vi "W7X2DPut_DAZ.vi"(4 "dimensions":i64[](array[numeric])=[1399090569999999999, -1], 5 "values":T1(array[cluster]), 6 "pulse_length":dbl, 7 "Unit":string, 8 "sample period":dbl, 9 "sample rate":u16, 10 "SigJSONbuffer":string, 11 "SigLabel":string) -> (0 "Parlog error out":errorcluster)   [LabVIEW 2014]
uses:
  <vilib>/httpClient/POSTBuffer.vi
  <vilib>/httpClient/LabVIEWHTTPClient.lvlib
panel:
  out "JSON string":string
  out "body":string
  out "headers":string
  out "body Parlog":string
  out "headers parms":string
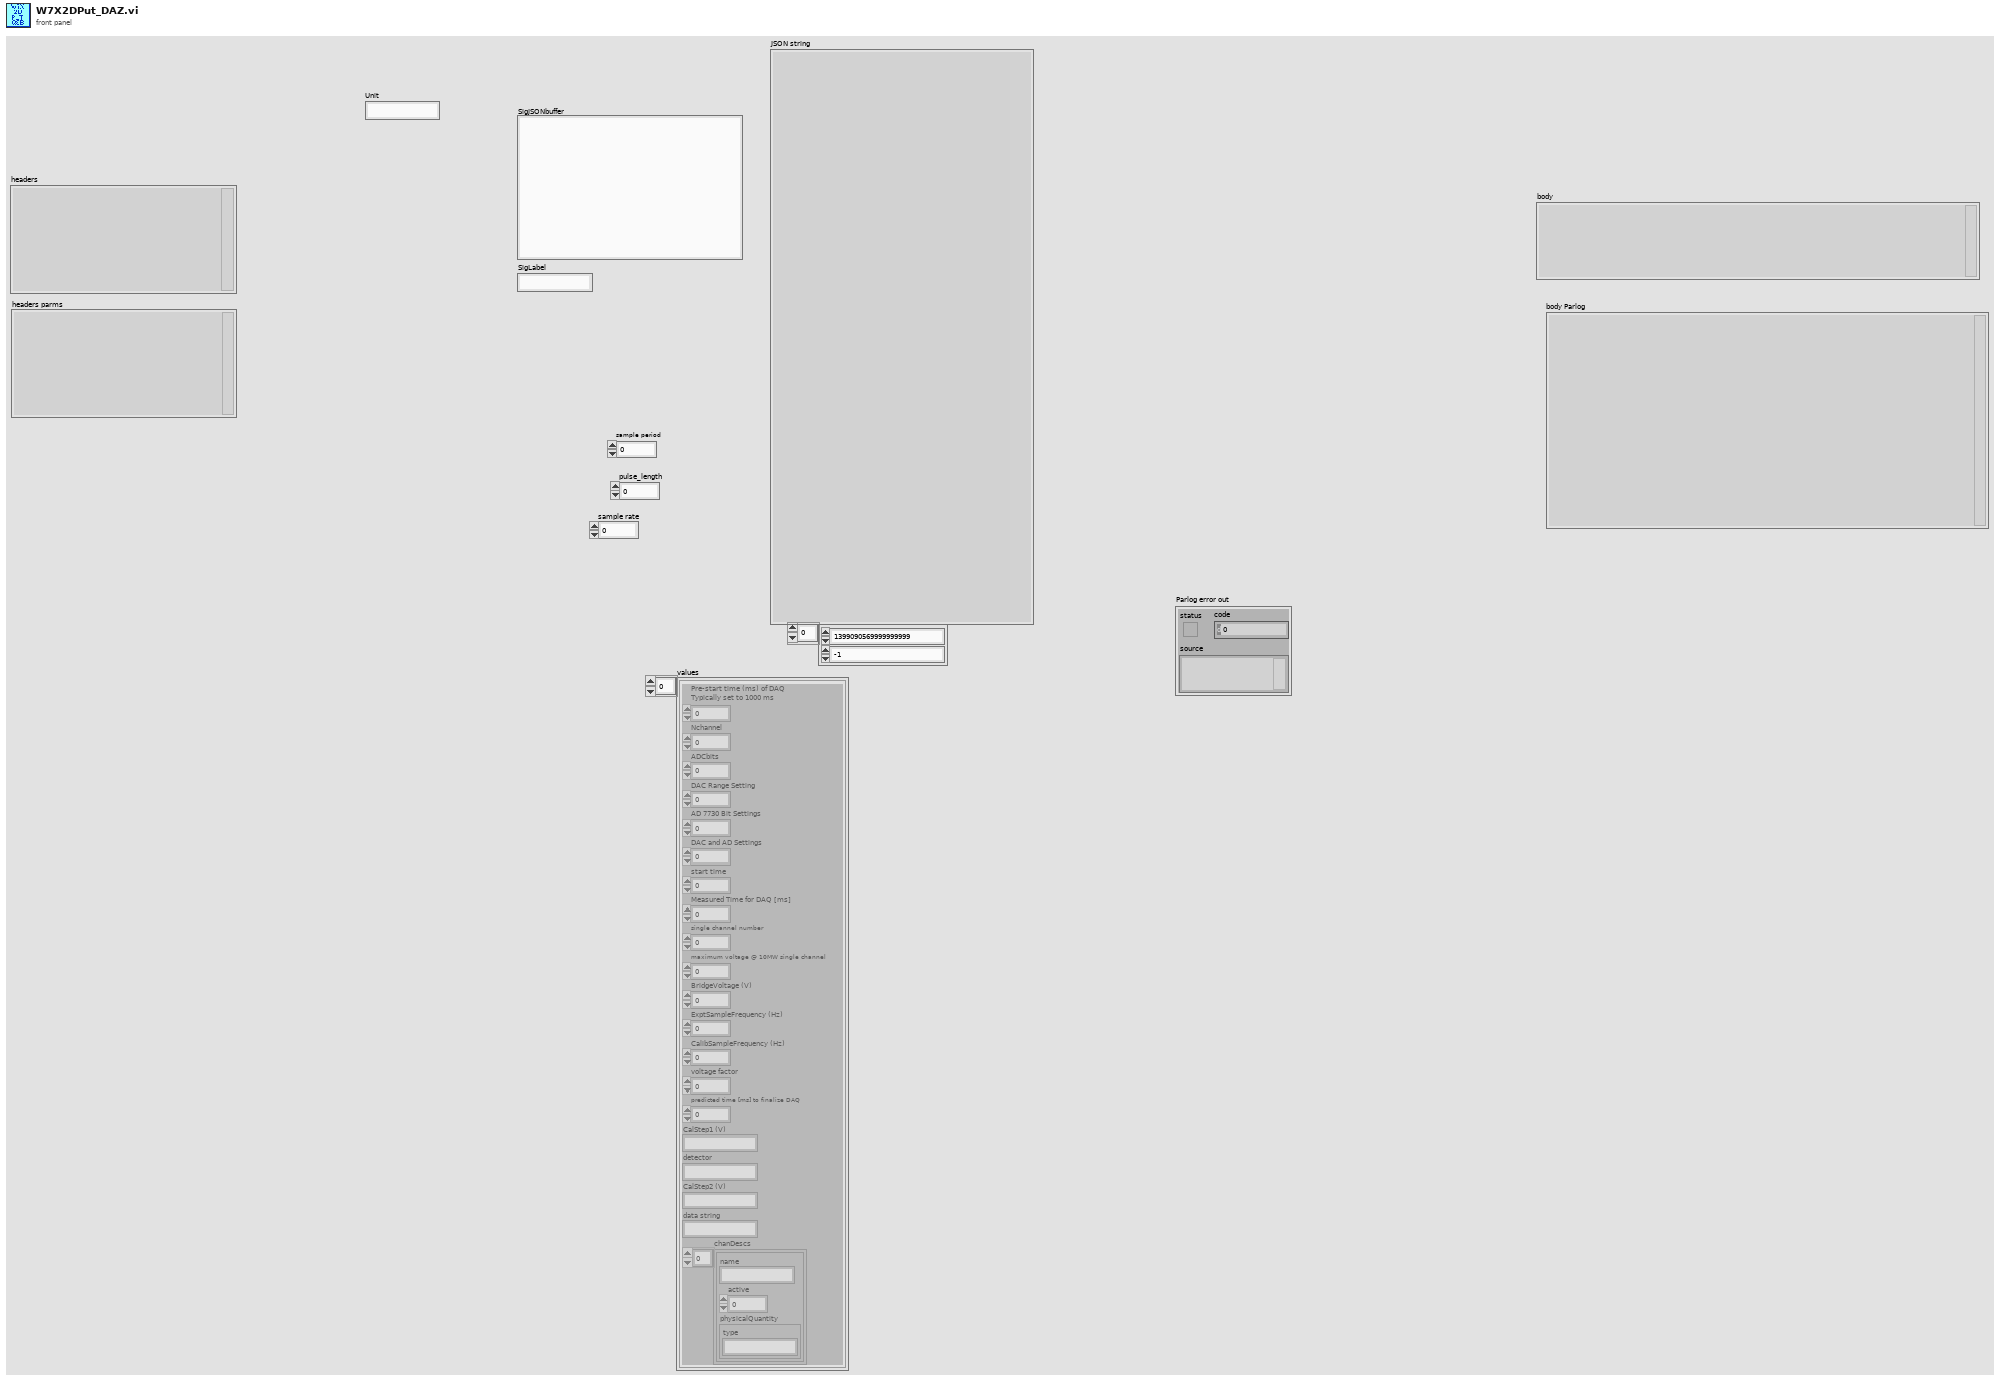
[diagram p1: front panel]
types:
  T1 = cluster{"Pre-start time (ms) of DAQ \nTypically set to 1000 ms":i32, "Nchannel":i16, "ADCbits":i16, "DAC Range Setting":u8, "AD 7730 Bit Settings":i32, "DAC and AD Settings":i32, "start time":i64, "Measured Time for DAQ [ms] ":u32, "single channel number":i64, "maximum voltage @ 10MW single channel":dbl, "BridgeVoltage (V)":sgl, "ExptSampleFrequency (Hz)":sgl, "CalibSampleFrequency (Hz)":sgl, "voltage factor":dbl, "predicted time [ms] to finalize DAQ":dbl, "CalStep1 (V)":string, "detector":string, "CalStep2 (V)":string, "data string":string, "chanDescs":cluster{"name":string, "active":i32, "physicalQuantity":cluster{"type":string}}[]}[]
  T2 = cluster{"Pre-start time (ms) of DAQ \nTypically set to 1000 ms":i32, "Nchannel":i16, "ADCbits":i16, "DAC Range Setting":u8, "AD 7730 Bit Settings":i32, "DAC and AD Settings":i32, "start time":i64, "Measured Time for DAQ [ms] ":u32, "single channel number":i64, "maximum voltage @ 10MW single channel":dbl, "BridgeVoltage (V)":sgl, "ExptSampleFrequency (Hz)":sgl, "CalibSampleFrequency (Hz)":sgl, "voltage factor":dbl, "predicted time [ms] to finalize DAQ":dbl, "CalStep1 (V)":string, "detector":string, "CalStep2 (V)":string, "data string":string, "chanDescs":cluster{"name":string, "active":i32, "physicalQuantity":cluster{"type":string}}[]}
  T3 = cluster{"name":string, "active":i32, "physicalQuantity":cluster{"type":string}}[]
  T4 = cluster{"name":string, "active":i32, "physicalQuantity":cluster{"type":string}}
  T5 = typedef "LabVIEWHTTPClient.lvlib/ClientHandle.ctl" = refnum<k1>
  T6 = cluster{"label":string, "values":cluster{"Pre-start time (ms) of DAQ \nTypically set to 1000 ms":i32, "Nchannel":i16, "ADCbits":i16, "DAC Range Setting":u8, "AD 7730 Bit Settings":i32, "DAC and AD Settings":i32, "start time":i64, "Measured Time for DAQ [ms] ":u32, "single channel number":i64, "maximum voltage @ 10MW single channel":dbl, "BridgeVoltage (V)":sgl, "ExptSampleFrequency (Hz)":sgl, "CalibSampleFrequency (Hz)":sgl, "voltage factor":dbl, "predicted time [ms] to finalize DAQ":dbl, "CalStep1 (V)":string, "detector":string, "CalStep2 (V)":string, "data string":string, "chanDescs":cluster{"name":string, "active":i32, "physicalQuantity":cluster{"type":string}}[]}[], "dimensions":i64[]}
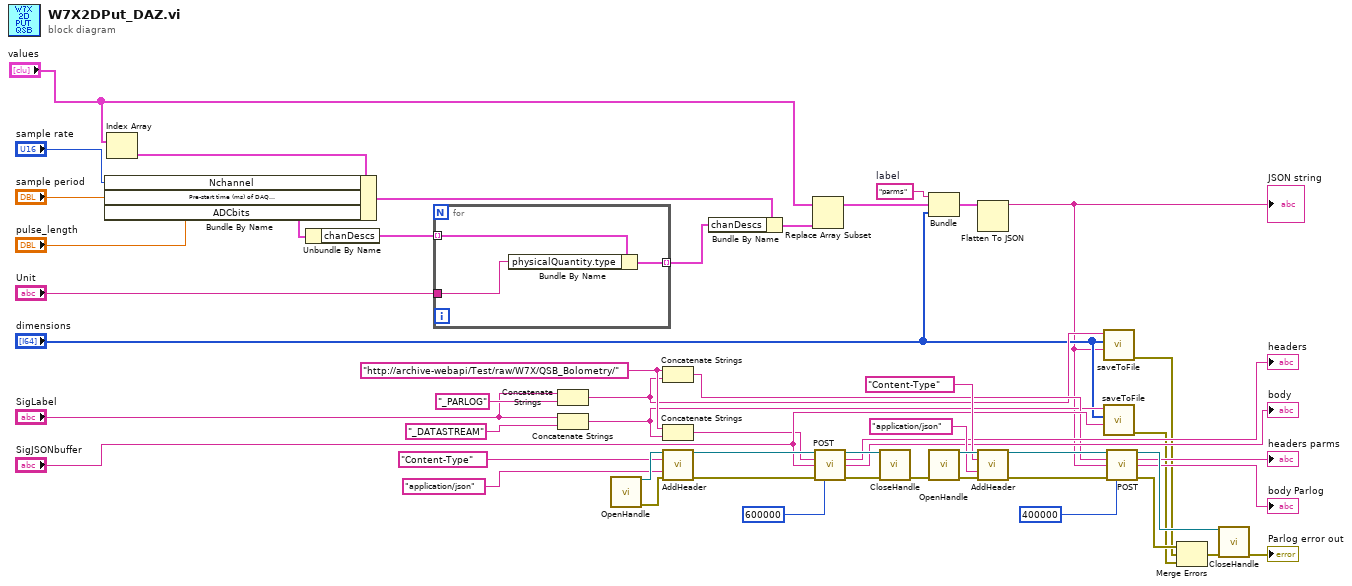
[diagram p0: block diagram]
diagram:
  w26 = "parms"  # label
  w10 = "http://archive-webapi/Test/raw/W7X/QSB_Bolometry/" ("url")
  n1 = Index Array(array="values") -> (element=w21:T2)  [unwired: 1 in]
  n2 = Bundle By Name(cluster=w21, "Nchannel"="sample rate", "Pre-start time (ms) of DAQ \nTypically set to 1000 ms"="sample period", "ADCbits"="pulse_length") -> (w18:T2)
  n3 = Unbundle By Name(w18) -> ("chanDescs"=w17:T3)
  n4 = for {
    tunnel: w17 -> [w54] mode=indexing
    tunnel: [w53] -> w16 mode=indexing
    tunnel: "Unit" -> [w52]
    n5 = Bundle By Name(cluster=w54, "physicalQuantity.type"=w52) -> (w53:T4)
  }
  n6 = Concatenate Strings("SigLabel", "_PARLOG" ("replace string (\"\")")) -> (w8:string)
  n7 = Concatenate Strings("SigLabel", "_DATASTREAM" ("string")) -> (w9:string)
  n8 = call <vilib>:"OpenHandle.vi"() -> ("client handle out"=w36:T5, "error out"=w35:errorcluster)  [unwired: 14 in]
  n9 = Concatenate Strings(w10, w8) -> (w11:string)
  n10 = Concatenate Strings(w10, w9) -> (w12:string)
  n11 = call <vilib>:"AddHeader.vi"("client handle"=w36, "header"="Content-Type", "value"="application/json", "error in (no error)"=w35) -> ("client handle out"=w34:T5, "error out"=w33:errorcluster)  [unwired: 10 in]
  n12 = Bundle By Name(cluster=w18, "chanDescs"=w16) -> (w20:T2)
  n13 = Replace Array Subset(array="values", new element=w20) -> (w19:T1)  [unwired: 1 in]
  n14 = call-poly <vilib>:"POST.vi"("client handle"=w34, "url"=w12, "buffer"="SigJSONbuffer", "error in (no error)"=w33, "timeout (10000)"=600000) -> ("client handle out"=w39:T5, "headers"=→"headers":string, "body"=→"body":string, "error out"=w38:errorcluster)  [unwired: 7 in]
  n15 = call <vilib>:"CloseHandle.vi"("client handle"=w39, "error in (no error)"=w38) -> ("error out"=w2:errorcluster)  [unwired: 13 in]
  n16 = Bundle("label"=w26, "values"=w19, "dimensions"="dimensions") -> (w25:T6)  [unwired: 1 in]
  n17 = call <vilib>:"OpenHandle.vi"("error in (no error)"=w2) -> ("client handle out"=w48:T5, "error out"=w47:errorcluster)  [unwired: 13 in]
  n18 = Flatten To JSON(anything=w25) -> (JSON string=w6:string)  [unwired: 2 in, 1 out]
  "JSON string" <- w6
  n19 = call <vilib>:"AddHeader.vi"("client handle"=w48, "header"="Content-Type", "value"="application/json", "error in (no error)"=w47) -> ("client handle out"=w46:T5, "error out"=w45:errorcluster)  [unwired: 10 in]
  n20 = call "saveToFile.vi"("SigJSONbuffer"=w6, "dimensions"="dimensions", "String"=w8) -> ("error out"=w4:errorcluster)  [unwired: 8 in]
  n21 = call "saveToFile.vi"("SigJSONbuffer"="SigJSONbuffer", "dimensions"="dimensions", "String"=w9) -> ("error out"=w3:errorcluster)  [unwired: 8 in]
  n22 = call-poly <vilib>:"POST.vi"("client handle"=w46, "url"=w11, "buffer"=w6, "error in (no error)"=w45, "timeout (10000)"=400000) -> ("client handle out"=w51:T5, "headers"=→"headers parms":string, "body"=→"body Parlog":string, "error out"=w50:errorcluster)  [unwired: 7 in]
  n23 = Merge Errors(w50, w4, w3) -> (w5:errorcluster)
  n24 = call <vilib>:"CloseHandle.vi"("client handle"=w51, "error in (no error)"=w5) -> ("error out"=→"Parlog error out":errorcluster)  [unwired: 13 in]
